vi "MatrixSwitchSingle.vi"(7 "Switch action":u16(ring) items=["Open", "Close"], 8 "error in (no error)":errorcluster, 9 "Matrix Y":i32=1 min=1 max=12 step=1, 10 "Matrix X":i32=1 min=1 max=12 step=1, 11 "Switching in":refnum<class "Switching.lvclass">) -> (0 "error out":errorcluster, 2 "command string":string, 3 "Switching out":refnum<class "Switching.lvclass">)   [LabVIEW 2013, in "Switching.lvclass"]
uses:
  Switching.lvclass
  Matrix_CommandsGlobal.vi
  InstrControl.lvclass
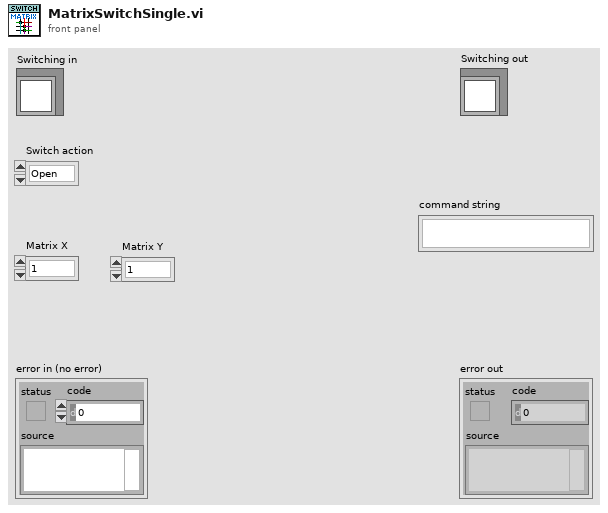
[diagram p1: front panel]
types:
  T1 = cluster{"Matrix address":string, "Instrument name":string, "Instrument type":u16, "Command \"Matrix Reset\"":string, "Command \"Connect Matrix Channels\"":string, "Command \"Disconnect Matrix Channels\"":string}
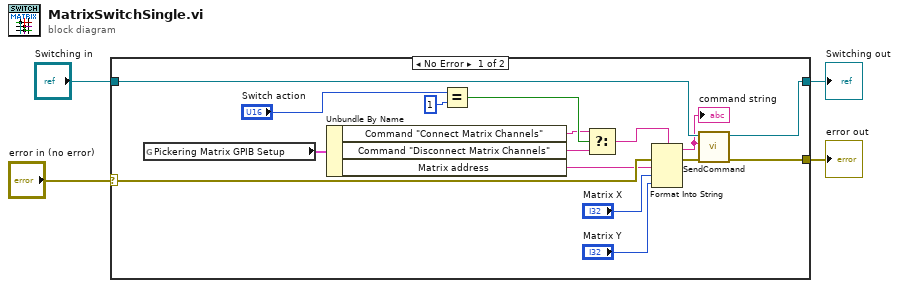
[diagram p0: block diagram]
diagram:
  n1 = case shown="No Error" "error in (no error)" {
    selector: "error in (no error)" -> [w18 w22]
    tunnel: [w14 w22] -> w3
    tunnel: [w13 w21] -> w1
    tunnel: "Switching in" -> [w17 w21]
    frame No Error {
      n2 = global read "Matrix_CommandsGlobal.vi" "Pickering Matrix GPIB Setup"() -> (w12:T1)
      n3 = Unbundle By Name(w12) -> ("Command \"Connect Matrix Channels\""=w8:string, "Command \"Disconnect Matrix Channels\""=w7:string, "Matrix address"=w5:string)
      n4 = Equal?(x="Switch action", y=1) -> (x = y?=w9:bool)
      n5 = Select(t=w8, s=w9, f=w7) -> (s? t:f=w6:string)
      n6 = Format Into String(format string=w6, error in=w18, w5, "Matrix X", "Matrix Y") -> (resulting string=w16:string, error out=w15:errorcluster)  [unwired: 1 in]
      "command string" <- w16
      n7 = call "SendCommand.vi"("error in (no error)"=w15, "Command string"=w16, "InstControl in"=w17) -> ("error out"=w14:errorcluster, "InstControl out"=w13:refnum<class "Switching.lvclass">)  [unwired: 7 in]
    }
    frame Error {
    }
  }
  "error out" <- w3
  "Switching out" <- w1
